vi "data stream main.vi"(11 "dataStream":T1) -> ()   [LabVIEW 2018]
uses:
  type defs/data stream data.ctl
  supporting VIs/polymorphic VIs/de-queue for data stream.vi
  supporting VIs/polymorphic VIs/enqueue for data stream.vi
  supporting VIs/polymorphic VIs/enqueue for data processor.vi
  supporting VIs/polymorphic VIs/release data stream queue.vi
types:
  T1 = typedef "data stream data.ctl" = cluster{"params":cluster{"Stream":cluster{"reader name":string, "RT IP address":string, "writer name":string, "stream buffer size":i32}}, "vars":cluster{"data stream":refnum<k21>}}
  T2 = typedef "Queues.ctl" = cluster{"messageHandler":refnum<queue>, "comms":refnum<queue>, "dataStream":refnum<queue>, "dataProcessor":refnum<queue>, "fileIO":refnum<queue>, "userInterface":refnum<queue>, "errors":refnum<queue>, "customCompressor":refnum<queue>}
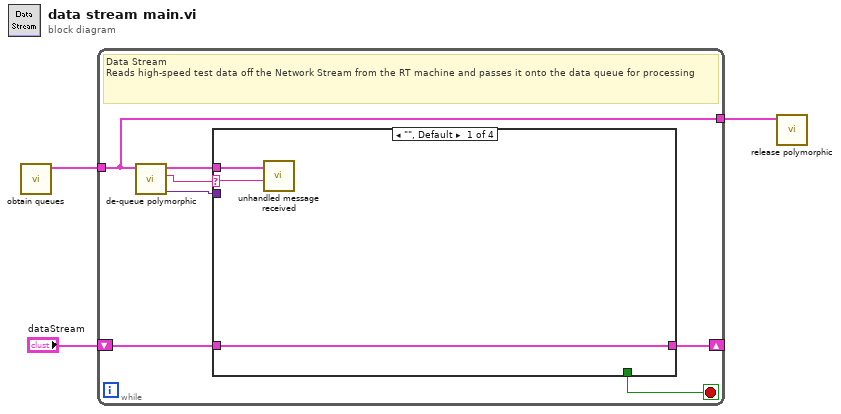
[diagram p0: block diagram]
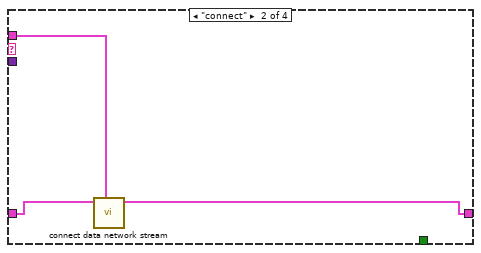
[diagram p2: hidden frame]
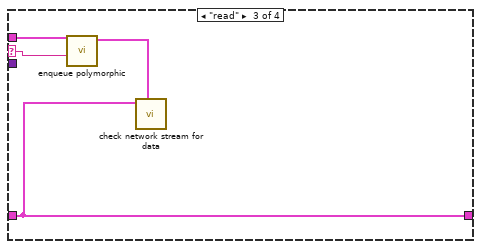
[diagram p3: hidden frame]
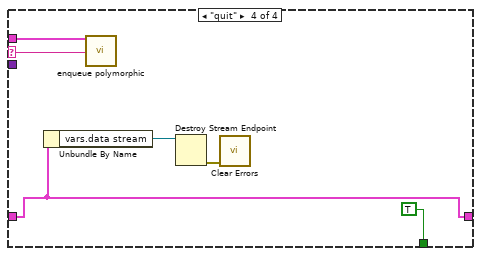
[diagram p4: hidden frame]
diagram:
  n1 = call "obtain queues.vi"() -> ("queues"=w2:T2)  [unwired: 11 in]
  n2 = while {
    tunnel: w2 -> [w4]
    shift-right: [w6] -> _
    shift-left: "dataStream" -> [w5]
    tunnel: [w4] -> w1
    stop <- w7 stop-if-true
    # "Data Stream\nReads high-speed test data off the Network Stream from the RT machine and passes it onto the data queue for processing"
    n3 = call-poly "de-queue polymorphic.vi"("Queues"=w4) -> ("data"=w8:variant, "message"=w9:string, "Queues out"=w10:T2)  [unwired: 8 in]
    n4 = case shown="\"\", Default" w9 {
      selector: w9 -> [w11 _ w18 w25]
      tunnel: w10 -> [w12 w14 w19 w26]
      tunnel: w8 -> [_ _ _ _]
      tunnel: [_ _ _ TRUE] -> w7
      tunnel: [w13 w15 w20 w23] -> w6
      tunnel: w5 -> [w13 w16 w20 w23]
      frame "", Default {
        n5 = call "unhandled message received.vi"("unhandledMessage"=w11, "queues"=w12) -> ()  [unwired: 10 in]
      }
      frame "connect" {
        n6 = call "connect data network stream.vi"("Queues"=w14, "dataStream in"=w16) -> ("dataStream out"=w15:T1)  [unwired: 9 in]
      }
      frame "read" {
        n7 = call-poly "enqueue polymorphic.vi"("message"=w18, "Queues"=w19) -> ("Queues out"=w17:T2)  [unwired: 9 in]
        n8 = call "check network stream for data.vi"("Queues in"=w17, "dataStream"=w20) -> ()  [unwired: 10 in]
      }
      frame "quit" {
        n9 = Unbundle By Name(w23) -> ("vars.data stream"=w22:refnum<k21>)
        n10 = call-poly "enqueue polymorphic.vi"("message"=w25, "Queues"=w26) -> ()  [unwired: 9 in, 1 out]
        n11 = Destroy Stream Endpoint(11:w22) -> (0:w21:errorcluster)  [unwired: 1 in]
        n12 = call <vilib>:"Clear Errors.vi"("error in (no error)"=w21) -> ()  [unwired: 5 in, 2 out]
      }
    }
  }
  n13 = call-poly "release polymorphic.vi"("Queues"=w1) -> ()  [unwired: 11 in]
